vi "ArmConstants.vi"() -> ()   [LabVIEW 2018]
panel:
  in  "Degrees/Tick":dbl=0.01
  in  "StartAngle":dbl=-60.0
  in  "ArmLength":dbl=48.0
  in  "RotationHeight":dbl=40.5
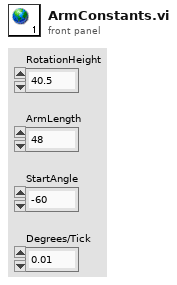
[diagram p1: front panel]
diagram:
